vi "MOV_Exclamation.vi"(0 "System no.":i32=1 min=1 max=4 step=1, 2 "Axes to move":string[](array[string]), 3 "Position values":dbl[](array[numeric]) format="%.6f", 4 "No.of digits":i16=4, 5 "error in":errorcluster) -> (19 "error out":errorcluster)   [LabVIEW 2020]
doc: "Moves specified axes to specified absolute positions and allows setting a new target position during the move without the move being interrupted. Use SCT.vi to set the cycle time for a periodic send. See user manual for details. No. of digits is the number of digits after the decimal point in the position value(s) that will be sent.\n\nC-887, F-206, M-8X0: Only for GCS syntax version = GCS 1.0 (Check with CSV?.vi. If CSV?.vi is not supported, syntax version is GCS 1.0). Axes to move can be X,Y,Z,U,V,W. For compatibility, calls MOV.vi for GCS 2.0 or higher. In this case, parameter 0x19001900 must be set to 1 (SPA.vi), see controller user manual for details."
uses:
  Controller names.ctl
  Syntax.ctl
  Global1.vi
  Global2 (Array).vi
panel:
  # "Moves stage and allows setting a new target position during\nmove. Use SCT.vi to set cycle time for periodic send."
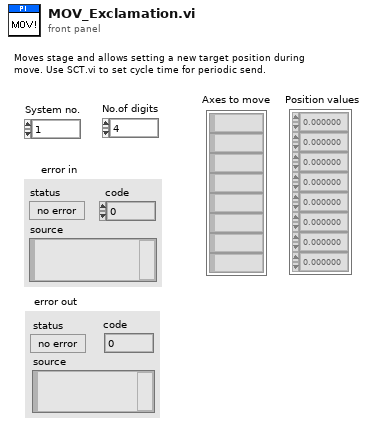
[diagram p1: front panel]
types:
  T1 = typedef "Syntax.ctl" = enum16{"GCS 1.0", "GCS 2.0", "GCS 3.0"}
  T2 = typedef "Controller names.ctl" = enum16{"None", "Analog", "C-702", "C-413", "C-414", "C-843", "C-843.PM", "C-844", "C-848", "C-865", "C-866", "C-867", "C-877", "C-880", "C-884", "C-885", "C-886", "C-887", "C-891", "E-135", "E-516", "E-517", "E-518", "E-709", "E-710", "E-712", "E-725", "E-727", "E-753", "E-754", "E-755", "E-761", "E-816", "E-861", "E-870", "E-871", "E-872", "E-873", "E-874", "F-206", "HydraPollux", "M-840", "M-850", "M-8X0", "Mercury", "Mercury_GCS", "PI_GCS2"}
  T3 = cluster{"Conn. axes":string[], "Controller name":T2}[]
  T4 = cluster{"Conn. axes":string[], "Controller name":T2}
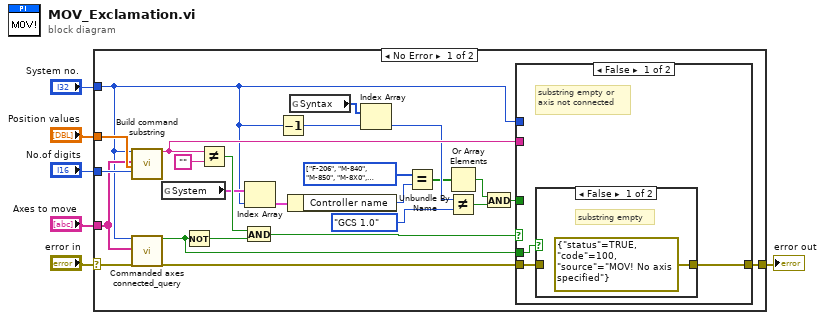
[diagram p0: block diagram]
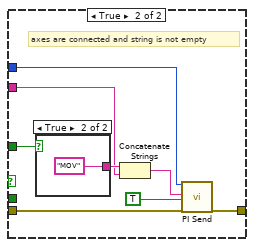
[diagram p3: hidden frame]
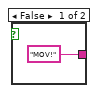
[diagram p4: hidden frame]
diagram:
  n1 = case shown="No Error" "error in" {
    selector: "error in" -> [w8 w47]
    tunnel: [w31 w47] -> w6
    tunnel: "Position values" -> [w28 _]
    tunnel: "No.of digits" -> [w27 _]
    tunnel: "System no." -> [w9 _]
    tunnel: "Axes to move" -> [w25 _]
    frame No Error {
      w17 = T2[] [enum."F-206", enum."M-840", enum."M-850", enum."M-8X0", enum."C-887"] items=["None", "Analog", "C-702", "C-413", "C-414", "C-843", "C-843.PM", "C-844", "C-848", "C-865", "C-866", "C-867", "C-877", "C-880", "C-884", "C-885", "C-886", "C-887", "C-891", "E-135", "E-516", "E-517", "E-518", "E-709", "E-710", "E-712", "E-725", "E-727", "E-753", "E-754", "E-755", "E-761", "E-816", "E-861", "E-870", "E-871", "E-872", "E-873", "E-874", "F-206", "HydraPollux", "M-840", "M-850", "M-8X0", "Mercury", "Mercury_GCS", "PI_GCS2"]
      n2 = call "Build command substring.vi"("System no."=w9, "Affected axes"=w25, "Parameters"=w28, "No. of digits"=w27) -> ("Command substring"=w29:string)  [unwired: 3 in, 12 out]
      n3 = call "Commanded axes connected_query.vi"("System no."=w9, "Commanded axes"=w25, "error in"=w8) -> ("Controller error"=w23:bool, "error out"=w26:errorcluster)  [unwired: 1 in, 14 out]
      n4 = global read "Global2 (Array).vi" "System"() -> (w14:T3)
      n5 = Not(x=w23) -> (.not. x?=w22:bool)
      n6 = Not Equal?(x=w29, y="") -> (x != y?=w24:bool)
      n7 = And(x=w24, y=w22) -> (x .and. y?=w21:bool)
      n8 = Index Array(array=w14, index=w9) -> (element=w15:T4)
      n9 = Decrement(x=w9) -> (x-1=w19:i32)
      n10 = Unbundle By Name(w15) -> ("Controller name"=w16:T2)
      n11 = global read "Global1.vi" "Syntax"() -> (w20:T1[])
      n12 = Index Array(array=w20, index=w19) -> (element=w18:T1)
      n13 = Equal?(x=w17, y=w16) -> (x = y?=w12:bool[])
      n14 = Or Array Elements(Boolean array=w12) -> (logical OR=w11:bool)
      n15 = Not Equal?(x=w18, y=Syntax."GCS 1.0") -> (x != y?=w13:bool)
      n16 = And(x=w11, y=w13) -> (x .and. y?=w10:bool)
      n17 = case shown="False" w21 {
        tunnel: w29 -> [_ w43]
        tunnel: [w34 w39] -> w31
        tunnel: w26 -> [w32 w40]
        tunnel: w23 -> [w33 _]
        tunnel: w9 -> [_ w38]
        tunnel: w10 -> [_ w37]
        frame False {
          # "substring empty or \naxis not connected"
          n18 = case shown="False" w33 {
            tunnel: [errorcluster {"status"=TRUE, "code"=100, "source"="MOV! No axis specified"} ("error out") w36] -> w34
            tunnel: w32 -> [_ w36]
            frame False {
              # "substring empty"
            }
            frame True {
              # "commanded axis \nnot connected"
            }
          }
        }
        frame True {
          # "axes are connected and string is not empty"
          n19 = case shown="True" w37 {
            tunnel: ["MOV!" "MOV"] -> w44
            frame False {
            }
            frame True {
            }
          }
          n20 = Concatenate Strings(w44, w43) -> (w41:string)
          n21 = call "PI Send.vi"("System no."=w38, "String to send"=w41, "Attach termination char.?"=TRUE ("Attach Linefeed?"), "error in"=w40) -> ("error out"=w39:errorcluster)  [unwired: 2 in, 13 out]
        }
      }
    }
    frame Error {
    }
  }
  "error out" <- w6
